vi "WaitForAsyncReturnData.vi"(8 "error in (no error)":errorcluster, 10 "timeout in ms (-1)":i32=-1, 11 "SMO":refnum<class "SMO.lvclass">) -> (0 "error out":errorcluster, 2 "Process Notification":T1, 3 "SMO out":refnum<class "SMO.lvclass">)   [LabVIEW 2021, in "smo.lvlib" / "SMO.lvclass"]
uses:
  SMO.lvclass
  Typedefs/Process Error Notification--Cluster.ctl
  SMO.lvclass/SMO.ctl
panel:
  # "For instructions on how to use the JKI State Machine Objects, examples and video tutorials, visit:\nhttp://jki.net/state-machine-objects/\n\nJKI State Machine Objects™\nhttp://jki.net/state-machine-objects/\nCopyright (C) 2005-2015, JKI <info@jki.net>\nALL RIGHTS RESERVED"
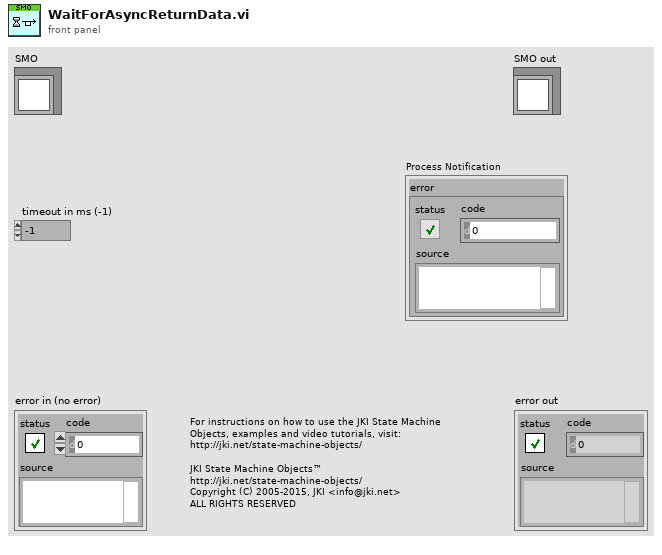
[diagram p1: front panel]
types:
  T1 = typedef "smo.lvlib/SMO.lvclass/Process Error Notification--Cluster.ctl" = cluster{"error":errorcluster}
  T2 = typedef "smo.lvlib/SMO.lvclass/PrivateData--Ref.ctl" = refnum<data-value>
  T3 = typedef "smo.lvlib/SMO.lvclass/PrivateData--Cluster.ctl" = cluster{"Parent Call":T4, "Registered Processes":T5[], "Sync Notifier":refnum<notifier>, "Process Error Notifier":refnum<notifier>, "Protected Events":T6, "Public Events":T7, "SMO State":T8, "[Attributes]":variant, "Launcher Close":refnum<notifier>, "Caller Watchdog":refnum<queue>, "Accessibility":T9, "NbStaticDependencies":u32}
  T4 = typedef "smo.lvlib/SMO.lvclass/Parent Call--Enum.ctl" = enum16{"Allows parent to run", "Does not request parent to run"}
  T5 = typedef "smo.lvlib/SMO.lvclass/RegisteredProcessData--Cluster.ctl" = cluster{"Name":string, "Static VI Ref":refnum<vi>, "Running":bool, "NotifierRef":u32}
  T6 = typedef "smo.lvlib/SMO.lvclass/Protected Events.ctl" = cluster{"StopProcesses":refnum<user-event>, "AbortProcesses":refnum<user-event>, "Config Changed":refnum<user-event>, "Dependency":refnum<user-event>}
  T7 = typedef "smo.lvlib/SMO.lvclass/Public Events.ctl" = cluster{"Error":refnum<user-event>, "State":refnum<user-event>, "Reserve State":refnum<user-event>}
  T8 = typedef "smo.lvlib/SMO.lvclass/SMOState --Enum.ctl" = enum16{"unknown", "Created", "Started", "Stopped"}
  T9 = typedef "smo.lvlib/SMO.lvclass/Accessibility--Cluster.ctl" = cluster{"Lock Key":string, "Reserve State":T10}
  T10 = typedef "smo.lvlib/SMO.lvclass/Reserve State--Enum.ctl" = enum16{"Unreserved", "Reserved", "Self-locked"}
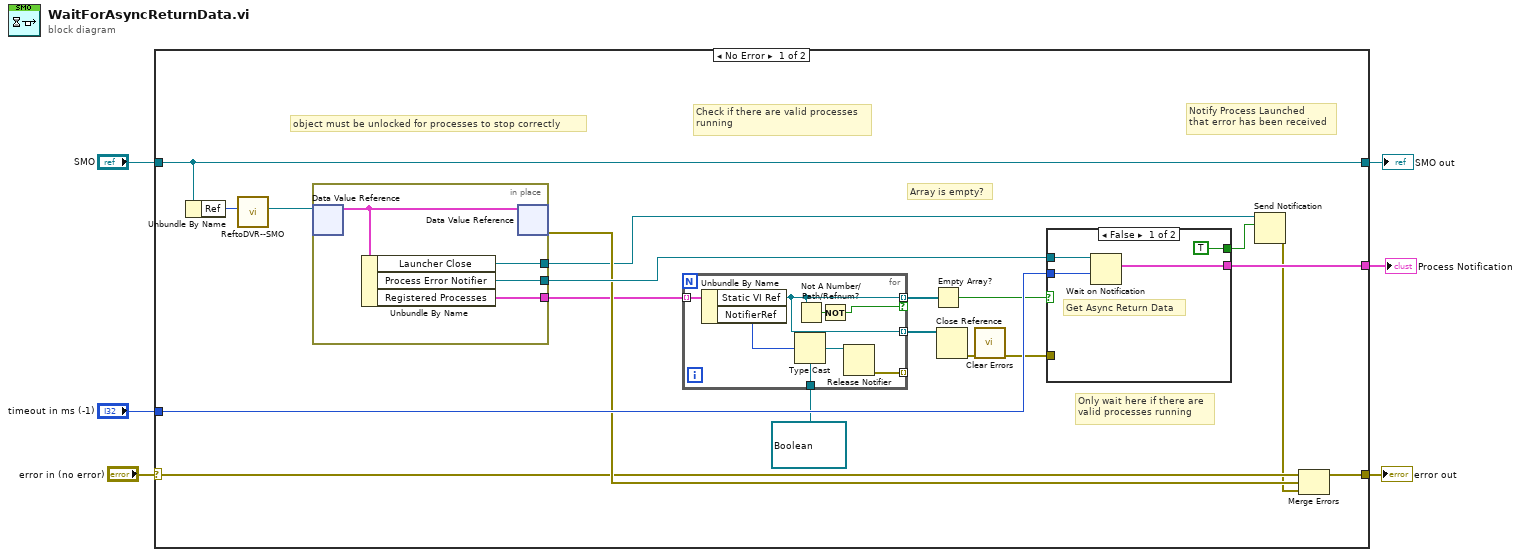
[diagram p0: block diagram]
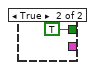
[diagram p2: hidden frame]
diagram:
  n1 = case shown="No Error" "error in (no error)" {
    selector: "error in (no error)" -> [w21 w44]
    tunnel: "timeout in ms (-1)" -> [w24 _]
    tunnel: [w22 w44] -> w5
    tunnel: "SMO" -> [w7 w43]
    tunnel: [w7 w43] -> w2
    tunnel: [w18 _] -> w1
    frame No Error {
      # "object must be unlocked for processes to stop correctly"
      # "Notify Process Launched\nthat error has been received"
      # "Check if there are valid processes\nrunning"
      # "Array is empty?"
      # "Only wait here if there are\nvalid processes running"
      n2 = Unbundle By Name(w7) -> ("Ref"=w9:u32)
      n3 = call "ReftoDVR--SMO.vi"("Ref"=w9) -> ("Ref"=w8:T2)  [unwired: 10 in]
      n4 = in-place {
        in-place-border: [w28] -> w25
        in-place-border: [w27] -> w20
        in-place-border: [w26] -> w17
        n5 = in-place-dvr #1(w8) -> (w29:T3)  [unwired: 1 out]
        n6 = Unbundle By Name(w29) -> ("Launcher Close"=w26:refnum<notifier>, "Process Error Notifier"=w28:refnum<notifier>, "Registered Processes"=w27:T5[])
        n7 = in-place-dvr #1(w29) -> (w23:errorcluster)  [unwired: 1 out]
      }
      n8 = for {
        tunnel: w20 -> [w35] mode=indexing
        tunnel: [w34] -> w14 mode=indexing if=w36
        tunnel: [w34] -> w11 mode=indexing
        tunnel: refnum<notifier> refnum ("notifier") -> [w32]
        tunnel: [w30] -> _ mode=indexing
        n9 = Unbundle By Name(w35) -> ("Static VI Ref"=w34:refnum<vi>, "NotifierRef"=w33:u32)
        n10 = Type Cast(type=w32, x=w33) -> (*(type *) &x=w31:refnum<notifier>)
        n11 = Not A Number/Path/Refnum?(number/path/refnum=w34) -> (NaN/Path/Refnum?=w37:bool)
        n12 = Not(x=w37) -> (.not. x?=w36:bool)
        n13 = Release Notifier(notifier=w31) -> (error out=w30:errorcluster)  [unwired: 2 in, 2 out]
      }
      n14 = Empty Array?(array=w14) -> (empty?=w19:bool)
      n15 = Close Reference(reference=w11) -> (error out=w12:errorcluster)  [unwired: 1 in]
      n16 = call <vilib>:"Clear Errors.vi"("error in (no error)"=w12) -> ("error out"=w13:errorcluster)  [unwired: 5 in, 1 out]
      n17 = case shown="False" w19 {
        tunnel: w24 -> [w41 _]
        tunnel: [w39 _] -> w18
        tunnel: w25 -> [w40 _]
        tunnel: [TRUE ("ignore previous (F)") TRUE ("ignore previous (F)")] -> w16
        tunnel: w13 -> [_ _]
        frame False {
          # "Get Async Return Data"
          n18 = Wait on Notification(notifier=w40, timeout in ms (-1)=w41) -> (notification=w39:T1)  [unwired: 2 in, 3 out]
        }
        frame True {
        }
      }
      n19 = Send Notification(notification=w16, notifier=w17) -> (error out=w15:errorcluster)  [unwired: 1 in, 1 out]
      n20 = Merge Errors(w21, w23, w15) -> (w22:errorcluster)
    }
    frame Error {
    }
  }
  "SMO out" <- w2
  "error out" <- w5
  "Process Notification" <- w1
